vi "_Return App Info.vi"(8 "error in (no error)":errorcluster, 11 "App Refnum in":refnum<vi>) -> (0 "error out":errorcluster, 2 "App Refnum for Opening VI":refnum<vi>, 5 "App Info":T1)   [LabVIEW 2017, in "CSM_ExampleBrowser.lvlib"]
uses:
  CSM_ExampleBrowser.lvlib
  <vilib>/addons/analyzer/_analyzerctrls.llb/VIAnCtl Analysis App Info.ctl
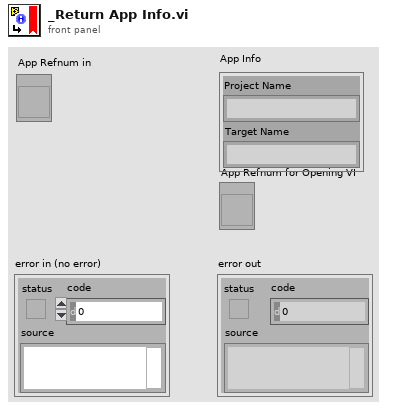
[diagram p1: front panel]
types:
  T1 = typedef "VIAnCtl Analysis App Info.ctl" = cluster{"Project Name":string, "Target Name":string}
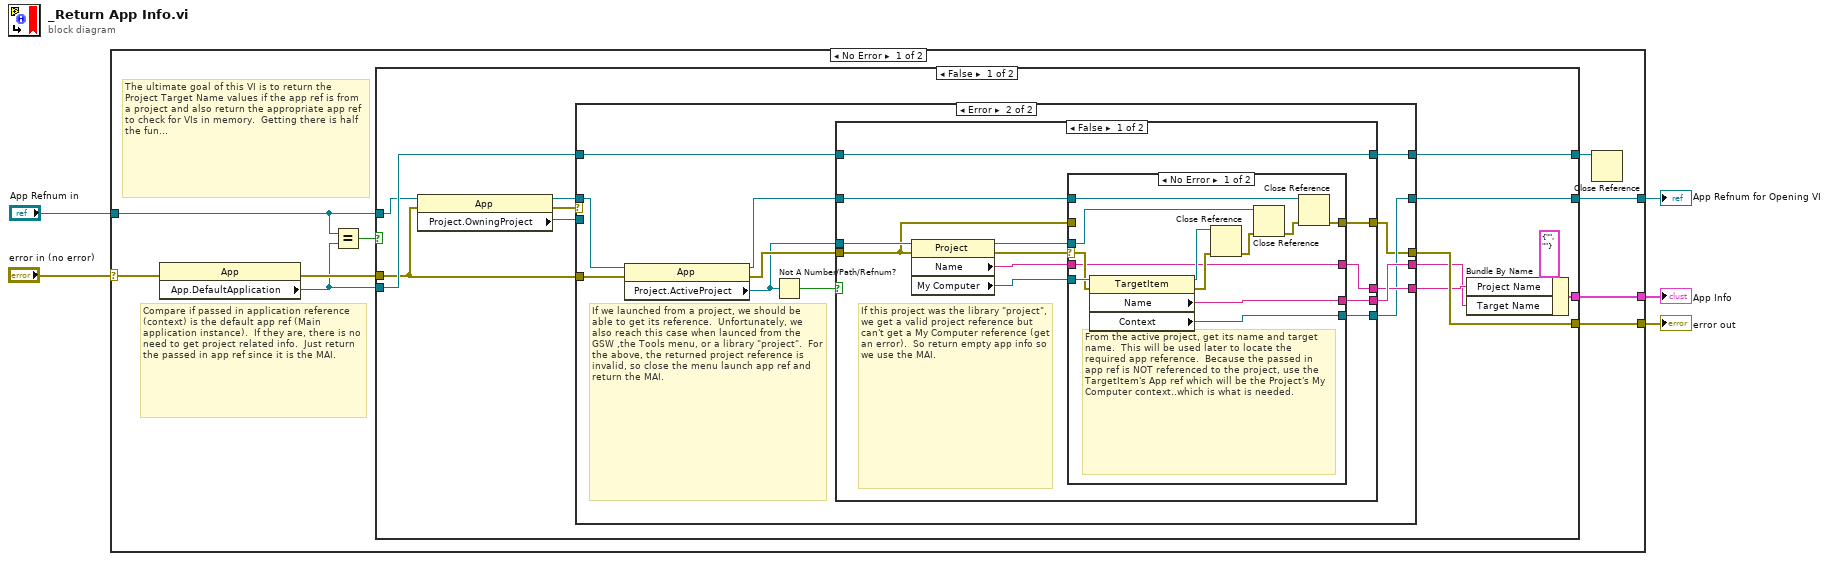
[diagram p0: block diagram]
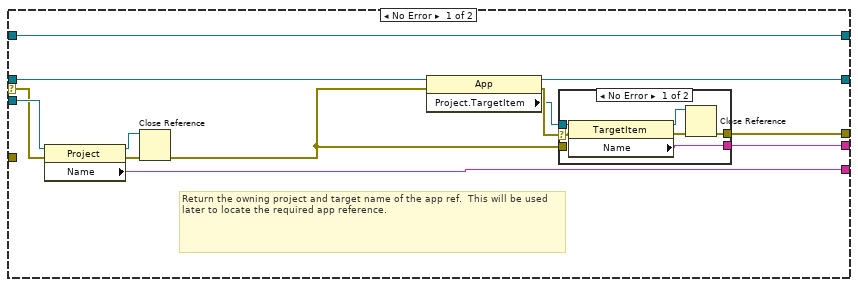
[diagram p2: hidden frame]
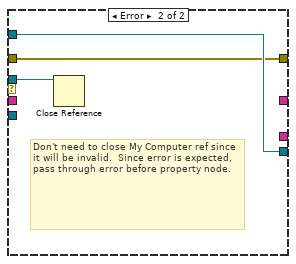
[diagram p4: hidden frame]
diagram:
  n1 = case shown="No Error" "error in (no error)" {
    selector: "error in (no error)" -> [w14 w93]
    tunnel: "App Refnum in" -> [w9 _]
    tunnel: [w12 w93] -> w3
    tunnel: [w11 _] -> w2
    tunnel: [w10 _] -> w1
    frame No Error {
      # "Compare if passed in application reference (context) is the default app ref (Main application instance).  If they are, there is no need to get project related info.  Just return the passed in app ref since it is the MAI."
      # "The ultimate goal of this VI is to return the Project Target Name values if the app ref is from a project and also return the appropriate app ref to check for VIs in memory.  Getting there is half the fun..."
      n2 = property class="App"(error in=w14) -> (error out=w13:errorcluster, "App.DefaultApplication"=w8:refnum<vi>)  [unwired: 1 in, 1 out]
      n3 = Equal?(x=w9, y=w8) -> (x = y?=w7:bool)
      n4 = case shown="False" w7 {
        tunnel: w13 -> [w15 w90]
        tunnel: [w27 w90] -> w12
        tunnel: [w26 w92] -> w11
        tunnel: [w25 _] -> w10
        tunnel: w9 -> [w19 w92]
        tunnel: w8 -> [w21 w91]
        tunnel: [w20 w91] -> w6
        frame False {
          n5 = property class="App"(reference=w19, error in=w15) -> (reference out=w17:refnum<vi>, error out=w16:errorcluster, "Project.OwningProject"=w18:refnum<vi>)
          n6 = case shown="Error" w16 {
            selector: w16 -> [w29 _]
            tunnel: [w40 w52] -> w27
            tunnel: [w39 w53] -> w26
            tunnel: [w33 w55] -> w23
            tunnel: [w32 w56] -> w22
            tunnel: w18 -> [w31 _]
            tunnel: w17 -> [w30 w58]
            tunnel: w15 -> [_ w59]
            tunnel: w21 -> [w28 w49]
            tunnel: [w28 w48] -> w20
            frame No Error {
              # "Return the owning project and target name of the app ref.  This will be used later to locate the required app reference."
              n7 = property class="Project"(reference=w31, error in=w29) -> (reference out=w37:refnum<vi>, error out=w38:errorcluster, "Name"=w33:string)
              n8 = Close Reference(reference=w37, error in (no error)=w38) -> (error out=w34:errorcluster)
              n9 = property class="App"(reference=w30, error in=w34) -> (reference out=w39:refnum<vi>, error out=w36:errorcluster, "Project.TargetItem"=w35:refnum<vi>)
              n10 = case shown="No Error" w36 {
                selector: w36 -> [w43 _]
                tunnel: w35 -> [w46 _]
                tunnel: [w42 w47] -> w40
                tunnel: [w41 _] -> w32
                tunnel: w34 -> [_ w47]
                frame No Error {
                  n11 = property class="TargetItem"(reference=w46, error in=w43) -> (reference out=w44:refnum<vi>, error out=w45:errorcluster, "Name"=w41:string)
                  n12 = Close Reference(reference=w44, error in (no error)=w45) -> (error out=w42:errorcluster)
                }
                frame Error {
                }
              }
            }
            frame Error {
              # "If we launched from a project, we should be able to get its reference.  Unfortunately, we also reach this case when launced from the GSW ,the Tools menu, or a library \"project\".  For the above, the returned project reference is invalid, so close the menu launch app ref and return the MAI."
              n13 = property class="App"(reference=w58, error in=w59) -> (reference out=w54:refnum<vi>, error out=w57:errorcluster, "Project.ActiveProject"=w51:refnum<vi>)
              n14 = Not A Number/Path/Refnum?(number/path/refnum=w51) -> (NaN/Path/Refnum?=w50:bool)
              n15 = case shown="False" w50 {
                tunnel: w57 -> [w60 w89]
                tunnel: [w69 _] -> w56
                tunnel: [w62 _] -> w55
                tunnel: w54 -> [w68 w87]
                tunnel: [w67 w88] -> w53
                tunnel: [w66 w89] -> w52
                tunnel: w51 -> [w65 _]
                tunnel: w49 -> [w61 w88]
                tunnel: [w61 w87] -> w48
                frame False {
                  # "If this project was the library \"project\", we get a valid project reference but can't get a My Computer reference (get an error).  So return empty app info so we use the MAI."
                  n16 = property class="Project"(reference=w65, error in=w60) -> (reference out=w71:refnum<vi>, error out=w64:errorcluster, "Name"=w63:string, "My Computer"=w70:refnum<vi>)
                  n17 = case shown="No Error" w64 {
                    selector: w64 -> [w73 _]
                    tunnel: w71 -> [w83 w86]
                    tunnel: w70 -> [w82 _]
                    tunnel: [w78 _] -> w69
                    tunnel: w68 -> [w77 w85]
                    tunnel: [w76 w85] -> w67
                    tunnel: [w74 w84] -> w66
                    tunnel: w63 -> [w72 _]
                    tunnel: [w72 _] -> w62
                    tunnel: w60 -> [_ w84]
                    frame No Error {
                      # "From the active project, get its name and target name.  This will be used later to locate the required app reference.  Because the passed in app ref is NOT referenced to the project, use the TargetItem's App ref which will be the Project's My Computer context..which is what is needed."
                      n18 = property class="TargetItem"(reference=w82, error in=w73) -> (reference out=w81:refnum<vi>, error out=w80:errorcluster, "Name"=w78:string, "Context"=w76:refnum<vi>)
                      n19 = Close Reference(reference=w81, error in (no error)=w80) -> (error out=w79:errorcluster)
                      n20 = Close Reference(reference=w83, error in (no error)=w79) -> (error out=w75:errorcluster)
                      n21 = Close Reference(reference=w77, error in (no error)=w75) -> (error out=w74:errorcluster)
                    }
                    frame Error {
                      # "Don't need to close My Computer ref since it will be invalid.  Since error is expected, pass through error before property node."
                      n22 = Close Reference(reference=w86) -> ()  [unwired: 1 in, 1 out]
                    }
                  }
                }
                frame True {
                }
              }
            }
          }
          n23 = Bundle By Name(cluster=T1 {"Project Name"="", "Target Name"=""} ("App Info"), "Project Name"=w23, "Target Name"=w22) -> (w25:T1)
        }
        frame True {
          # "For the MAI, app info is not applicable."
        }
      }
      n24 = Close Reference(reference=w6) -> ()  [unwired: 1 in, 1 out]
    }
    frame Error {
    }
  }
  "error out" <- w3
  "App Refnum for Opening VI" <- w2
  "App Info" <- w1
